vi "Periodic Tasks.vi"() -> ()   [LabVIEW 2011]
doc: "This VI runs in parallel to other tasks. It can contain as many user-defined periodic loops as you need. These can carry out PID or other sorts of timed response."
uses:
  <vilib>/Rock Robotics/SystemInterfaces/Utilities/FPGA_UtilitiesLED State.ctl
  <vilib>/Rock Robotics/SystemInterfaces/Utilities/FPGA_UtilitiesLED Source.ctl
  Robot Global Data.vi
  <vilib>/Rock Robotics/WPI/Relay/WPI_RelayValue.ctl
panel:
  in  "Reset Ball":bool
  in  "Home Speed":dbl=0.4
  out "Auton Recording":bool
  in  "Turn on Record":bool
  in  "Auton Array":dbl[][](array[numeric])
  out "Ramp ACT Pot":dbl
  out "Right Rate":dbl
  out "Right Direction":bool
  out "Right Distance":dbl
  out "Shooter Encoder Distance":dbl
  out "Shooter Direction":bool
  out "Shooter Encoder Rate":dbl
  out "Left Rate":dbl
  out "Gyro Rate":dbl
  out "Gyro Angle":dbl
  out "Left Direction":bool
  out "Left Distance":dbl
  # "Auton Recording"
  # "Sensor Feedback"
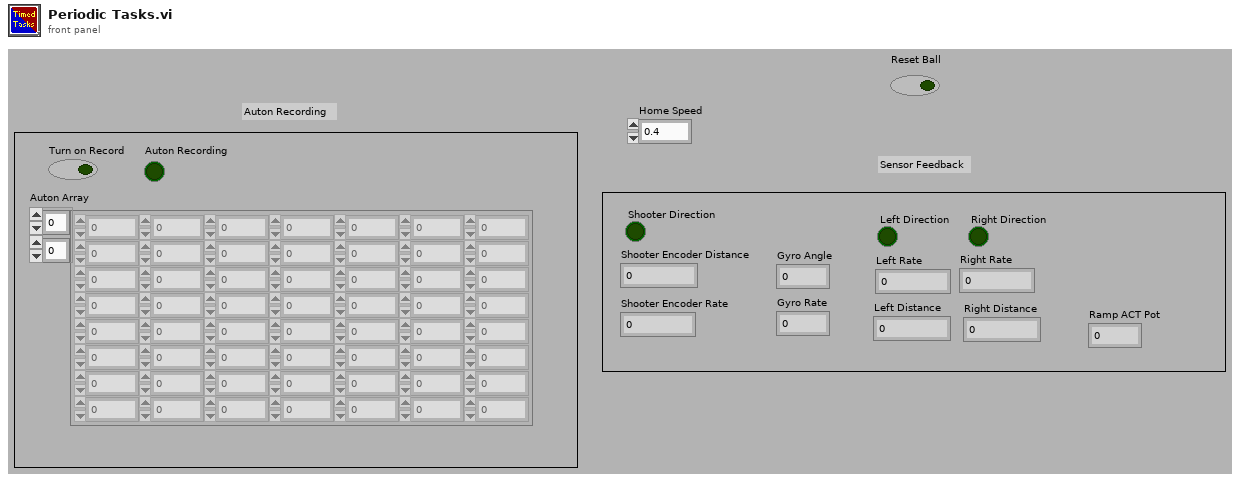
[diagram p1: front panel]
types:
  T1 = typedef "WPI_RelayValue.ctl" = enum16{"Off", "On", "Forward", "Reverse"}
  T2 = typedef "WPI_AnalogChannelDevRef.ctl" = cluster{"DevStatus":errorcluster, "Analog Module":T3, "Analog Channel":T4}
  T3 = typedef "FPGA_TypedefAnalogModule.ctl" = enum16{"Analog Module 1", "Analog Module 2"}
  T4 = typedef "FPGA_AIChannel.ctl" = enum8{"AI 1", "AI 2", "AI 3", "AI 4", "AI 5", "AI 6", "AI 7", "AI 8", "Invalid"}
  T5 = typedef "WPI_EncoderDevRef.ctl" = cluster{"DevStatus":errorcluster, "EncoderIndex":T6, "CounterIndex":T7, "DistancePerCount":dbl, "Decoding Type":T8}
  T6 = typedef "FPGA_EncoderIdx.ctl" = enum8{"Enc 0", "Enc 1", "Enc 2", "Enc 3", "Invalid"}
  T7 = typedef "FPGA_CounterCtrSystemIndex.ctl" = enum8{"Ctr 0", "Ctr 1", "Ctr 2", "Ctr 3", "Ctr 4", "Ctr 5", "Ctr 6", "Ctr 7", "Invalid"}
  T8 = typedef "WPI_EncoderType.ctl" = enum16{"1x", "2x", "4x"}
  T9 = typedef "WPI_GyroDevRef.ctl" = cluster{"DevStatus":errorcluster, "Analog Module":T3, "Analog Channel":T4, "Offset":dbl, "Gain (VoltsPerDegree/Second)":dbl}
  T10 = typedef "WPI_RelayDevRef.ctl" = cluster{"DevStatus":errorcluster, "Relay Channel":T11, "Digital Module":T12, "Relay Direction":T13}
  T11 = typedef "FPGA_DIORelayChannel.ctl" = enum8{"Relay 1", "Relay 2", "Relay 3", "Relay 4", "Relay 5", "Relay 6", "Relay 7", "Relay 8", "Invalid"}
  T12 = typedef "FPGA_TypedefDigitalModule.ctl" = enum16{"Digital Module 1", "Digital Module 2"}
  T13 = typedef "WPI_RelayDirection.ctl" = enum16{"Both directions", "Forward only", "Reverse only"}
  T14 = typedef "FPGA_UtilitiesLED State.ctl" = enum16{"Off", "On", "Toggle"}
  T15 = typedef "FPGA_UtilitiesLED Source.ctl" = enum16{"User LED", "FPGA LED"}
  T16 = cluster{"Left Drive Output":dbl, "Right Drive Output":dbl, "Ramp Actuator Output":dbl, "Harvester Output":dbl, "Conveyer Output":dbl, "Turret Rotation":dbl, "Shooter Output":dbl}
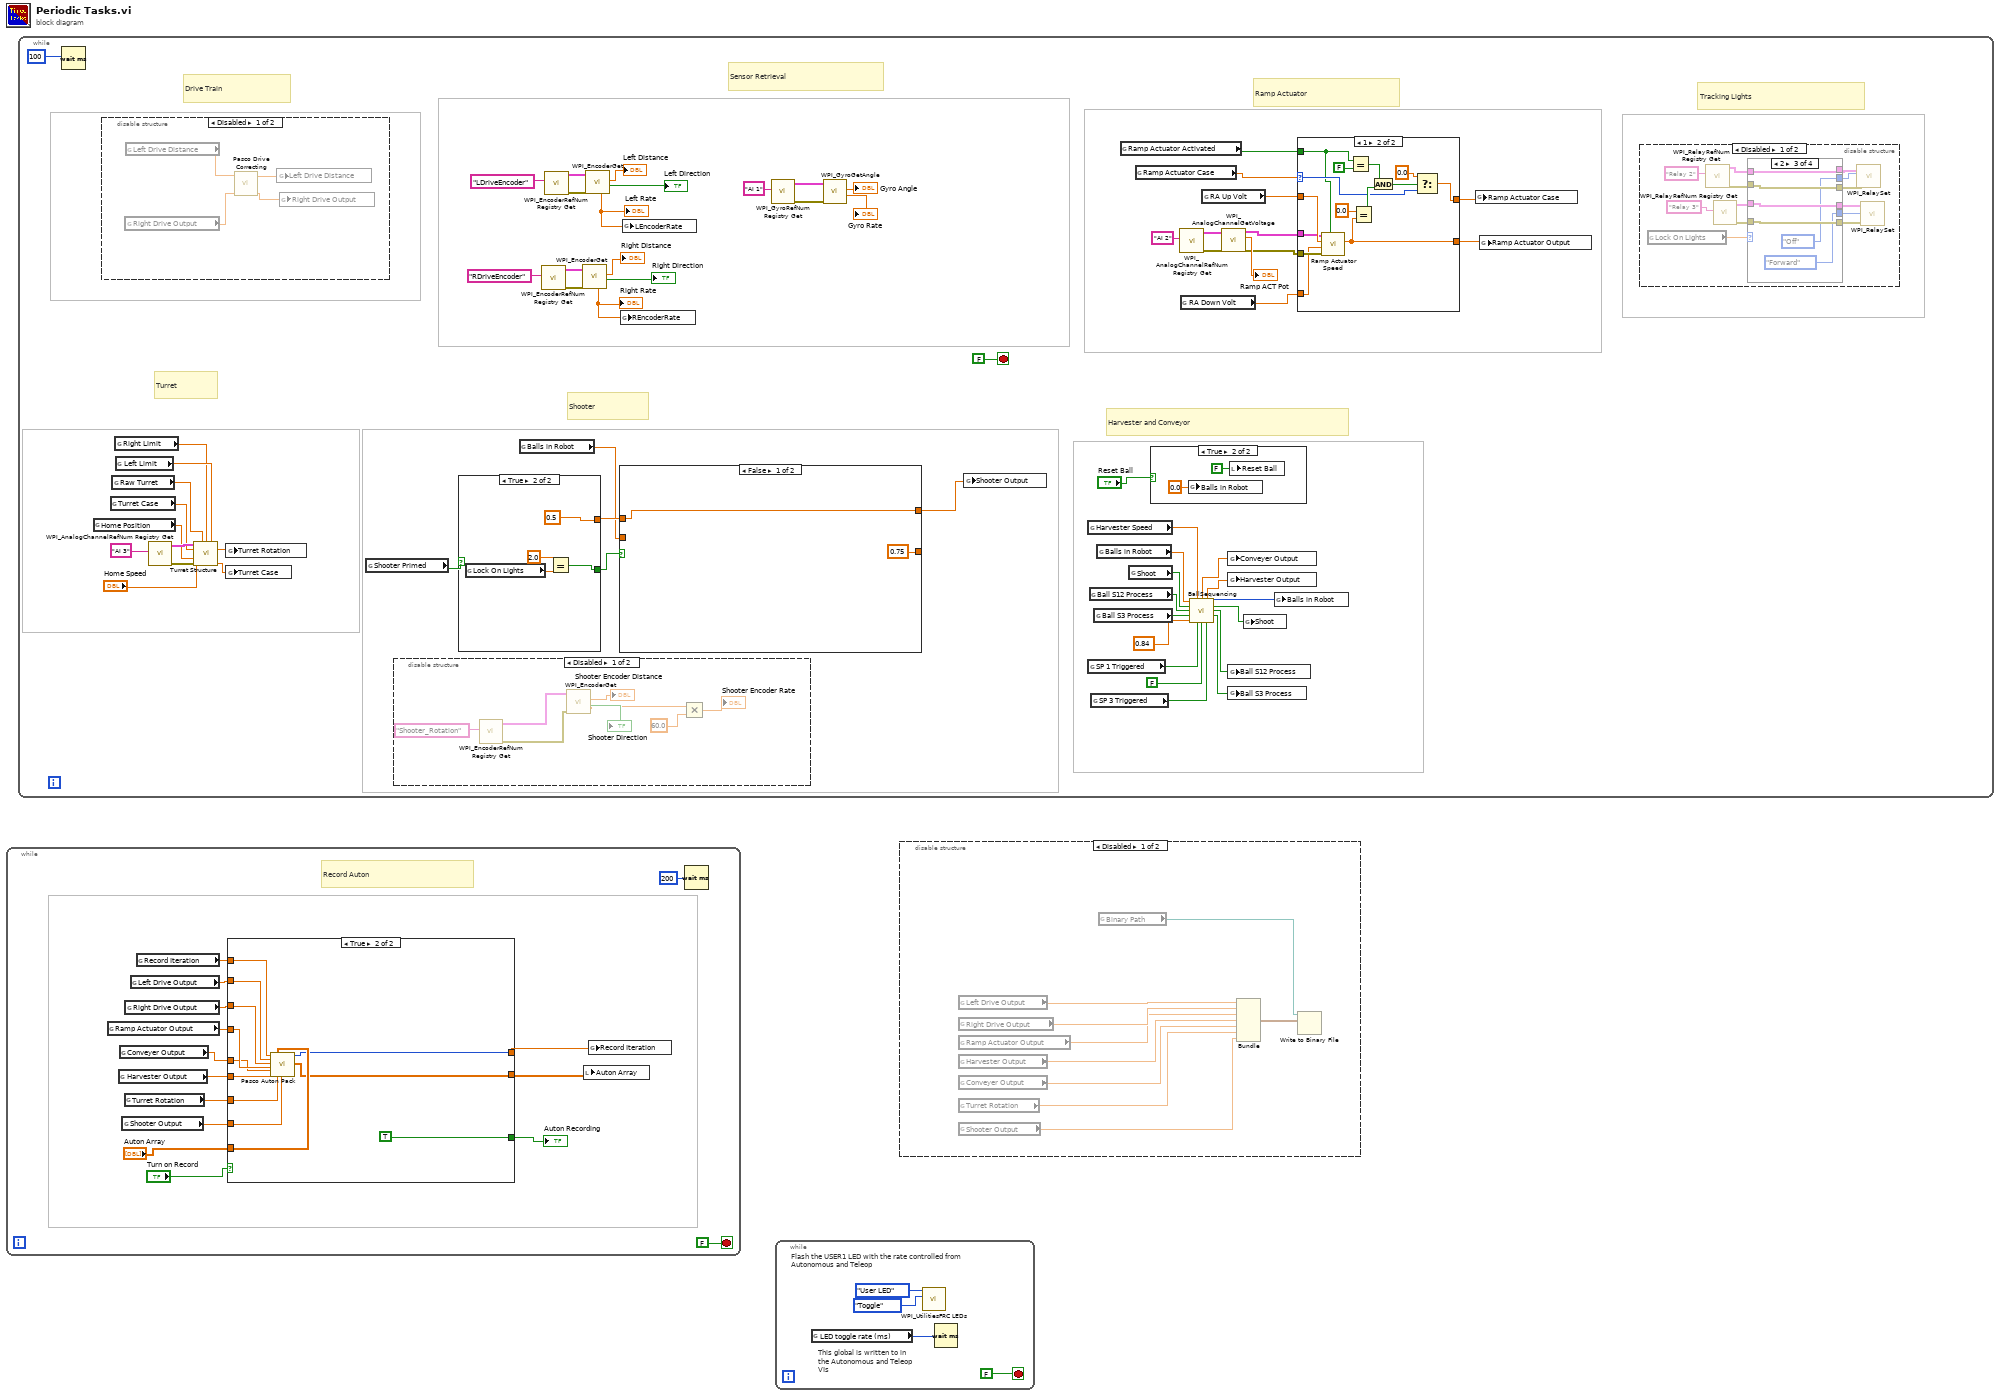
[diagram p0: block diagram]
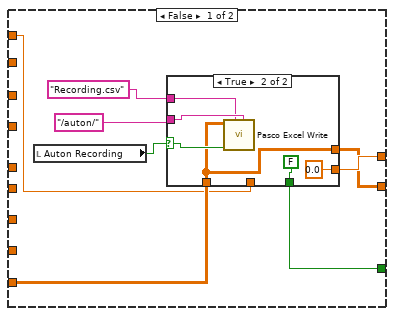
[diagram p2: hidden frame]
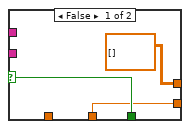
[diagram p3: hidden frame]
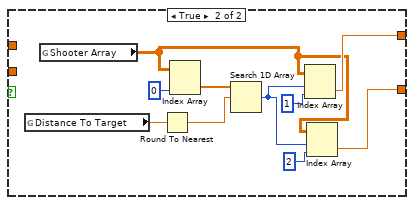
[diagram p5: hidden frame]
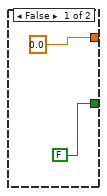
[diagram p6: hidden frame]
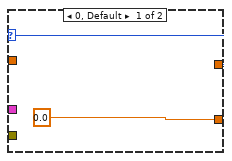
[diagram p8: hidden frame]
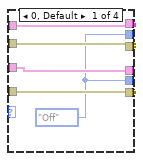
[diagram p9: hidden frame]
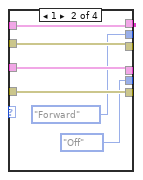
[diagram p10: hidden frame]
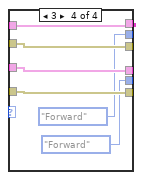
[diagram p11: hidden frame]
diagram:
  n1 = while {
    stop <- FALSE stop-if-true
    # "Record Auton"
    n2 = global read "Robot Global Data.vi" "Ramp Actuator Output"() -> (w5:dbl)
    n3 = global read "Robot Global Data.vi" "Harvester Output"() -> (w7:dbl)
    n4 = global read "Robot Global Data.vi" "Conveyer Output"() -> (w6:dbl)
    n5 = global read "Robot Global Data.vi" "Shooter Output"() -> (w9:dbl)
    n6 = global read "Robot Global Data.vi" "Turret Rotation"() -> (w8:dbl)
    n7 = global read "Robot Global Data.vi" "Right Drive Output"() -> (w4:dbl)
    n8 = global read "Robot Global Data.vi" "Left Drive Output"() -> (w3:dbl)
    n9 = global read "Robot Global Data.vi" "Record Iteration"() -> (w2:dbl)
    n10 = case shown="True" "Turn on Record" {
      tunnel: w2 -> [w19 w44]
      tunnel: w3 -> [_ w43]
      tunnel: w4 -> [_ w42]
      tunnel: w5 -> [_ w41]
      tunnel: w6 -> [_ w40]
      tunnel: w7 -> [_ w39]
      tunnel: w8 -> [_ w38]
      tunnel: w9 -> [_ w37]
      tunnel: "Auton Array" -> [w20 w36]
      tunnel: [w16 w35] -> w12
      tunnel: [w17 w34] -> w13
      tunnel: [w18 TRUE] -> w14
      frame False {
        n11 = local read "Auton Recording"() -> (w21:bool)
        n12 = case shown="True" w21 {
          selector: w21 -> [w26 w31]
          tunnel: [w26 FALSE] -> w18
          tunnel: "/auton/" ("File Name") -> [_ w30]
          tunnel: "Recording.csv" ("Folder Location") -> [_ w29]
          tunnel: [w25 0.0 ("Record Iteration")] -> w17
          tunnel: w19 -> [w25 _]
          tunnel: w20 -> [_ w27]
          tunnel: [dbl[][] [] ("Auton Array") w27] -> w16
          frame False {
          }
          frame True {
            n13 = call "Pasco Excel Write.vi"("Folder Location"=w30, "File Name"=w29, "WriteToExcel"=w31, "2D data"=w27) -> ()  [unwired: 7 in, 1 out]
          }
        }
      }
      frame True {
        n14 = call "Pasco Auton Pack.vi"("Iterations"=w44, "Left Drive"=w43, "Right Drive"=w42, "RAMP ACT"=w41, "Conveyor"=w40, "Harvestor"=w39, "Auton Array"=w36, "Turret"=w38, "Shooter"=w37) -> ("Iteration Output"=w34:i32, "output array"=w35:dbl[][])  [unwired: 9 in]
      }
    }
    "Auton Recording" <- w14
    n15 = local write "Auton Array"(w12) -> ()
    n16 = global write "Robot Global Data.vi" "Record Iteration"(w13) -> ()
    n17 = Wait (ms)(milliseconds to wait=u32 200) -> ()  [unwired: 1 out]
  }
  n18 = while {
    stop <- FALSE stop-if-true
    # "Tracking Lights"
    # "Harvester and Conveyor"
    # "Shooter"
    # "Sensor Retrieval"
    # "Turret"
    # "Drive Train"
    # "Ramp Actuator"
    n19 = Wait (ms)(milliseconds to wait=u32 100) -> ()  [unwired: 1 out]
    n20 = global read "Robot Global Data.vi" "Home Position"() -> (w101:dbl)
    n21 = disable-structure shown="Disabled" {
      frame Disabled {
        n22 = global read "Robot Global Data.vi" "Right Drive Output"() -> (w182:dbl)
        n23 = global read "Robot Global Data.vi" "Left Drive Distance"() -> (w183:dbl)
        n24 = call "Pasco Drive Correcting.vi"("RightDriveOutput"=w182, "LeftDriveOutput"=w183) -> ("RightDriveOutput"=w180:dbl, "LeftDriveOutput"=w181:dbl)  [unwired: 8 in]
        n25 = global write "Robot Global Data.vi" "Left Drive Distance"(w181) -> ()
        n26 = global write "Robot Global Data.vi" "Right Drive Output"(w180) -> ()
      }
      frame Enabled {
      }
    }
    n27 = global read "Robot Global Data.vi" "Turret Case"() -> (w102:dbl)
    n28 = global read "Robot Global Data.vi" "Raw Turret"() -> (w100:dbl)
    n29 = global read "Robot Global Data.vi" "Right Limit"() -> (w83:dbl)
    n30 = global read "Robot Global Data.vi" "Left Limit"() -> (w84:dbl)
    n31 = call <vilib>:"WPI_AnalogChannelRefNum Registry Get.vi"("refnum name"="AI 3") -> ("error out"=w103:errorcluster, "AIDeviceRef"=w104:T2)  [unwired: 9 in]
    n32 = call "Turret Structure.vi"("AIDeviceRef"=w104, "Raw Turret"=w100, "upper limit"=w83, "lower limit"=w84, "Turret Case"=w102, "Home Speed"="Home Speed", "Home postion"=w101, "error in (no error)"=w103) -> ("Turret Output"=w99:dbl, "Turret Case Output"=w98:dbl)  [unwired: 6 in]
    n33 = global write "Robot Global Data.vi" "Turret Rotation"(w99) -> ()
    n34 = global write "Robot Global Data.vi" "Turret Case"(w98) -> ()
    n35 = global read "Robot Global Data.vi" "Shooter Primed"() -> (w70:bool)
    n36 = disable-structure shown="Disabled" {
      frame Disabled {
        n37 = call <vilib>:"WPI_EncoderRefNum Registry Get.vi"("refnum name"="Shooter_Rotation") -> ("error out"=w184:errorcluster, "EncoderDevRef"=w185:T5)  [unwired: 9 in]
        n38 = call <vilib>:"WPI_EncoderGet.vi"("error in (no error)"=w184, "EncoderDevRef"=w185) -> ("Direction"=→"Shooter Direction":bool, "Distance"=→"Shooter Encoder Distance":dbl, "Rate"=w188:dbl)  [unwired: 4 in, 3 out]
        n39 = Multiply(x=w188, y=60.0) -> (x*y=→"Shooter Encoder Rate":dbl)
      }
      frame Enabled {
      }
    }
    n40 = case shown="True" w70 {
      tunnel: [FALSE ("Shooter Primed") w122] -> w69
      tunnel: [0.0 0.5] -> w67
      frame False {
      }
      frame True {
        n41 = global read "Robot Global Data.vi" "Lock On Lights"() -> (w124:dbl)
        n42 = Equal?(x=2.0, y=w124) -> (x = y?=w122:bool)
      }
    }
    n43 = global read "Robot Global Data.vi" "Balls in Robot"() -> (w66:dbl)
    n44 = call <vilib>:"WPI_EncoderRefNum Registry Get.vi"("refnum name"="RDriveEncoder") -> ("error out"=w49:errorcluster, "EncoderDevRef"=w48:T5)  [unwired: 9 in]
    n45 = call <vilib>:"WPI_EncoderRefNum Registry Get.vi"("refnum name"="LDriveEncoder") -> ("error out"=w55:errorcluster, "EncoderDevRef"=w54:T5)  [unwired: 9 in]
    n46 = call <vilib>:"WPI_EncoderGet.vi"("error in (no error)"=w49, "EncoderDevRef"=w48) -> ("Direction"=→"Right Direction":bool, "Distance"=→"Right Distance":dbl, "Rate"=w45:dbl)  [unwired: 4 in, 3 out]
    "Right Rate" <- w45
    n47 = call <vilib>:"WPI_EncoderGet.vi"("error in (no error)"=w55, "EncoderDevRef"=w54) -> ("Direction"=→"Left Direction":bool, "Distance"=→"Left Distance":dbl, "Rate"=w51:dbl)  [unwired: 4 in, 3 out]
    "Left Rate" <- w51
    n48 = case shown="False" w69 {
      tunnel: [w109 w119] -> w68
      tunnel: w67 -> [w109 _]
      tunnel: w66 -> [_ _]
      tunnel: [0.75 w118] -> _
      frame False {
      }
      frame True {
        n49 = global read "Robot Global Data.vi" "Distance To Target"() -> (w115:dbl)
        n50 = global read "Robot Global Data.vi" "Shooter Array"() -> (w110:dbl[][])
        n51 = Round To Nearest(number=w115) -> (nearest integer value=w114:dbl)
        n52 = Index Array(array=w110, index (col)=0 ("disabled index (col)")) -> (element=w113:dbl[])  [unwired: 1 in]
        n53 = Search 1D Array(1D array=w113, element=w114) -> (index of element=w111:i32)  [unwired: 1 in]
        n54 = Index Array(array=w110, index (row)=w111, index (col)=1 ("disabled index (col)")) -> (element=w119:dbl)
        n55 = Index Array(array=w110, index (row)=w111, index (col)=2 ("disabled index (col)")) -> (element=w118:dbl)
      }
    }
    n56 = global write "Robot Global Data.vi" "REncoderRate"(w45) -> ()
    n57 = global write "Robot Global Data.vi" "LEncoderRate"(w51) -> ()
    n58 = call <vilib>:"WPI_GyroRefNum Registry Get.vi"("refnum name"="AI 1") -> ("error out"=w63:errorcluster, "GyroDevRef"=w64:T9)  [unwired: 9 in]
    n59 = call <vilib>:"WPI_GyroGetAngle.vi"("error in (no error)"=w63, "GyroDevRef"=w64) -> ("Angular Rate"=→"Gyro Rate":dbl, "Angle"=→"Gyro Angle":dbl)  [unwired: 6 in, 2 out]
    n60 = global write "Robot Global Data.vi" "Shooter Output"(w68) -> ()
    n61 = global read "Robot Global Data.vi" "Harvester Speed"() -> (w65:dbl)
    n62 = global read "Robot Global Data.vi" "SP 1 Triggered"() -> (w74:bool)
    n63 = global read "Robot Global Data.vi" "Ball S12 Process"() -> (w76:bool)
    n64 = global read "Robot Global Data.vi" "SP 3 Triggered"() -> (w73:bool)
    n65 = global read "Robot Global Data.vi" "Ball S3 Process"() -> (w75:bool)
    n66 = global read "Robot Global Data.vi" "Balls in Robot"() -> (w78:dbl)
    n67 = global read "Robot Global Data.vi" "Ramp Actuator Activated"() -> (w91:bool)
    n68 = global read "Robot Global Data.vi" "Shoot"() -> (w77:bool)
    n69 = global read "Robot Global Data.vi" "Ramp Actuator Case"() -> (w93:dbl)
    n70 = case shown="True" "Reset Ball" {
      frame False {
      }
      frame True {
        n71 = global write "Robot Global Data.vi" "Balls in Robot"(0.0 ("Balls in Robot")) -> ()
        n72 = local write "Reset Ball"(FALSE ("Reset Ball")) -> ()
      }
    }
    n73 = call <vilib>:"WPI_AnalogChannelRefNum Registry Get.vi"("refnum name"="AI 2") -> ("error out"=w89:errorcluster, "AIDeviceRef"=w90:T2)  [unwired: 9 in]
    n74 = global read "Robot Global Data.vi" "RA Down Volt"() -> (w96:dbl)
    n75 = call "BallSequencing.vi"("Balls In Robot"=w78, "Speed of Harvester"=w65, "Shoot"=w77, "Ball S12 Process"=w76, "Ball S3 Process"=w75, "Speed of Conveyor"=0.84, "SP 1 Triggered"=w74, "SP 2 Triggered"=FALSE, "SP 3 Triggered"=w73) -> ("Conveyer Output"=w79:dbl, "Harvester Output"=w80:dbl, "Balls In Robot Output"=w58:i32, "Shoot Output"=w57:bool, "Ball S12 Process Output"=w82:bool, "Ball S3 Process Output"=w81:bool)  [unwired: 1 in]
    n76 = global read "Robot Global Data.vi" "RA Up Volt"() -> (w95:dbl)
    n77 = call <vilib>:"WPI_AnalogChannelGetVoltage.vi"("error in (no error)"=w89, "AIDeviceRef"=w90) -> ("error out"=w86:errorcluster, "Voltage"=→"Ramp ACT Pot":dbl, "AIDeviceRef"=w87:T2)  [unwired: 7 in]
    n78 = global write "Robot Global Data.vi" "Conveyer Output"(w79) -> ()
    n79 = global write "Robot Global Data.vi" "Harvester Output"(w80) -> ()
    n80 = global write "Robot Global Data.vi" "Ball S12 Process"(w82) -> ()
    n81 = global write "Robot Global Data.vi" "Ball S3 Process"(w81) -> ()
    n82 = global write "Robot Global Data.vi" "Shoot"(w57) -> ()
    n83 = global write "Robot Global Data.vi" "Balls in Robot"(w58) -> ()
    n84 = case shown="1" w93 {
      selector: w93 -> [w128 w133]
      tunnel: w86 -> [_ w143]
      tunnel: w96 -> [_ w142]
      tunnel: w95 -> [_ w141]
      tunnel: [0.0 ("Ramp Actuator Ouput") w132] -> w94
      tunnel: w91 -> [_ w131]
      tunnel: [w128 w134] -> w92
      tunnel: w87 -> [_ w130]
      frame 0, Default {
      }
      frame 1 {
        n85 = call "Ramp Actuator Speed.vi"("Up to Down"=w131, "error in (no error)"=w143, "RA Down Volt"=w142, "RA Up Volt"=w141, "AIDeviceRef"=w130) -> ("Ramp Actuator Ouput"=w132:dbl)  [unwired: 6 in]
        n86 = Equal?(x=w131, y=FALSE) -> (x = y?=w138:bool)
        n87 = Equal?(x=0.0, y=w132) -> (x = y?=w139:bool)
        n88 = And(x=w138, y=w139) -> (x .and. y?=w136:bool)
        n89 = Select(t=0.0, s=w136, f=w133) -> (s? t:f=w134:dbl)
      }
    }
    n90 = global write "Robot Global Data.vi" "Ramp Actuator Case"(w92) -> ()
    n91 = global write "Robot Global Data.vi" "Ramp Actuator Output"(w94) -> ()
    n92 = disable-structure shown="Disabled" {
      frame Disabled {
        n93 = global read "Robot Global Data.vi" "Lock On Lights"() -> (w144:dbl)
        n94 = call <vilib>:"WPI_RelayRefNum Registry Get.vi"("refnum name"="Relay 2") -> ("error out"=w151:errorcluster, "RelayDevRef"=w153:T10)  [unwired: 9 in]
        n95 = call <vilib>:"WPI_RelayRefNum Registry Get.vi"("refnum name"="Relay 3") -> ("error out"=w148:errorcluster, "RelayDevRef"=w149:T10)  [unwired: 9 in]
        n96 = case shown="2" w144 {
          tunnel: [w161 w167 w173 w179] -> w154
          tunnel: w153 -> [w161 w167 w173 w179]
          tunnel: [w160 w166 w172 w178] -> w152
          tunnel: w151 -> [w160 w166 w172 w178]
          tunnel: [w159 w165 w171 w177] -> w150
          tunnel: w149 -> [w159 w165 w171 w177]
          tunnel: w148 -> [w158 w164 w170 w176]
          tunnel: [w158 w164 w170 w176] -> w147
          tunnel: [w157 WPI_RelayValue."Forward" ("RelayValue") WPI_RelayValue."Off" ("RelayValue") WPI_RelayValue."Forward" ("RelayValue")] -> w146
          tunnel: [w157 WPI_RelayValue."Off" ("RelayValue") WPI_RelayValue."Forward" ("RelayValue") WPI_RelayValue."Forward" ("RelayValue")] -> w145
          frame 0, Default {
            w157 = WPI_RelayValue."Off" ("RelayValue")
          }
          frame 1 {
          }
          frame 2 {
          }
          frame 3 {
          }
        }
        n97 = call <vilib>:"WPI_RelaySet.vi"("error in (no error)"=w152, "RelayValue"=w146, "RelayDevRef"=w154) -> ()  [unwired: 7 in, 2 out]
        n98 = call <vilib>:"WPI_RelaySet.vi"("error in (no error)"=w147, "RelayValue"=w145, "RelayDevRef"=w150) -> ()  [unwired: 7 in, 2 out]
      }
      frame Enabled {
      }
    }
  }
  n99 = while {
    stop <- FALSE stop-if-true
    # "This global is written to in the Autonomous and Teleop VIs"
    # "Flash the USER1 LED with the rate controlled from Autonomous and Teleop"
    n100 = global read "Robot Global Data.vi" "LED toggle rate (ms)"() -> (w192:u32)
    n101 = call <vilib>:"WPI_UtilitiesFRC LEDs.vi"("State"=FPGA_UtilitiesLED_State."Toggle", "LED Type"=FPGA_UtilitiesLED_Source."User LED") -> ()  [unwired: 1 in, 9 out]
    n102 = Wait (ms)(milliseconds to wait=w192) -> ()  [unwired: 1 out]
  }
  n103 = disable-structure shown="Disabled" {
    frame Disabled {
      n104 = global read "Robot Global Data.vi" "Left Drive Output"() -> (w204:dbl)
      n105 = global read "Robot Global Data.vi" "Right Drive Output"() -> (w203:dbl)
      n106 = global read "Robot Global Data.vi" "Ramp Actuator Output"() -> (w202:dbl)
      n107 = global read "Robot Global Data.vi" "Harvester Output"() -> (w201:dbl)
      n108 = global read "Robot Global Data.vi" "Conveyer Output"() -> (w200:dbl)
      n109 = global read "Robot Global Data.vi" "Turret Rotation"() -> (w199:dbl)
      n110 = global read "Robot Global Data.vi" "Shooter Output"() -> (w198:dbl)
      n111 = global read "Robot Global Data.vi" "Binary Path"() -> (w196:path)
      n112 = Bundle("Left Drive Output"=w204, "Right Drive Output"=w203, "Ramp Actuator Output"=w202, "Harvester Output"=w201, "Conveyer Output"=w200, "Turret Rotation"=w199, "Shooter Output"=w198) -> (w197:T16)  [unwired: 1 in]
      n113 = Write to Binary File(file (use dialog)=w196, data=w197) -> ()  [unwired: 4 in, 3 out]
    }
    frame Enabled {
    }
  }
